vi "rethinkdb_hashlib_sha256_hmac.vi"(10 "data":string="The quick brown fox jumps over the lazy dog", 11 "key":string="key") -> (3 "sha256":u32[](array[numeric]) format="%08x")   [LabVIEW 2017]
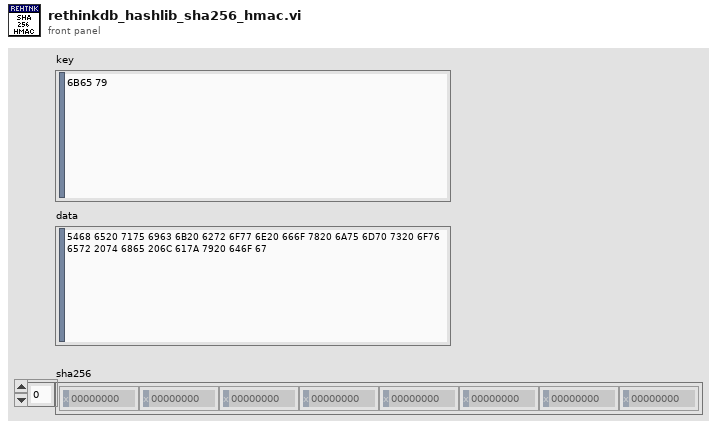
[diagram p1: front panel]
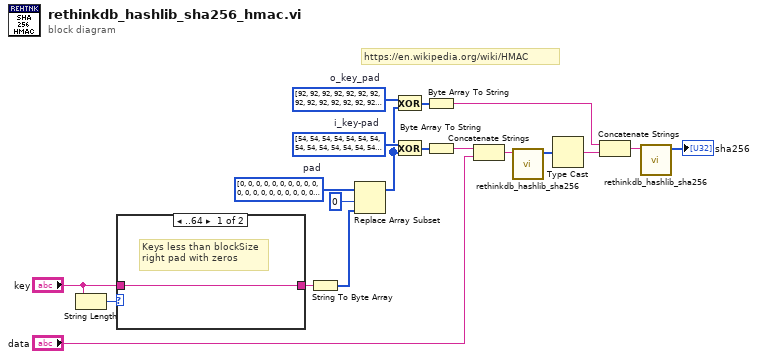
[diagram p0: block diagram]
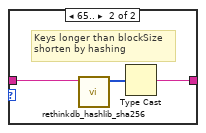
[diagram p2: hidden frame]
diagram:
  w8 = u8[] [0, 0, 0, 0, 0, 0, 0, 0, 0, 0, 0, 0, 0, 0, 0, 0, 0, 0, 0, 0, 0, 0, 0, 0, 0, 0, 0, 0, 0, 0, 0, 0, 0, 0, 0, 0, 0, 0, 0, 0, 0, 0, 0, 0, 0, 0, 0, 0, 0, 0, 0, 0, 0, 0, 0, 0, 0, 0, 0, 0, 0, 0, 0, 0]  # pad
  w10 = u8[] [92, 92, 92, 92, 92, 92, 92, 92, 92, 92, 92, 92, 92, 92, 92, 92, 92, 92, 92, 92, 92, 92, 92, 92, 92, 92, 92, 92, 92, 92, 92, 92, 92, 92, 92, 92, 92, 92, 92, 92, 92, 92, 92, 92, 92, 92, 92, 92, 92, 92, 92, 92, 92, 92, 92, 92, 92, 92, 92, 92, 92, 92, 92, 92]  # o_key_pad
  w9 = u8[] [54, 54, 54, 54, 54, 54, 54, 54, 54, 54, 54, 54, 54, 54, 54, 54, 54, 54, 54, 54, 54, 54, 54, 54, 54, 54, 54, 54, 54, 54, 54, 54, 54, 54, 54, 54, 54, 54, 54, 54, 54, 54, 54, 54, 54, 54, 54, 54, 54, 54, 54, 54, 54, 54, 54, 54, 54, 54, 54, 54, 54, 54, 54, 54]  # i_key-pad
  # "https://en.wikipedia.org/wiki/HMAC"
  n1 = String Length(string="key") -> (length=w12:i32)
  n2 = case shown="..64" w12 {
    tunnel: "key" -> [w20 w21]
    tunnel: [w20 w22] -> w7
    frame ..64 {
      # "Keys less than blockSize\nright pad with zeros"
    }
    frame 65.. {
      # "Keys longer than blockSize\nshorten by hashing"
      n3 = call "rethinkdb_hashlib_sha256.vi"("data"=w21) -> ("sha256"=w23:u32[])  [unwired: 10 in]
      n4 = Type Cast(x=w23) -> (*(type *) &x=w22:string)  [unwired: 1 in]
    }
  }
  n5 = String To Byte Array(string=w7) -> (unsigned byte array=w6:u8[])
  n6 = Replace Array Subset(array=w8, new element=w6, index=0) -> (w5:u8[])
  n7 = Exclusive Or(1:w5, 2:w10) -> (0:w15:u8[])
  n8 = Exclusive Or(1:w5, 2:w9) -> (0:w19:u8[])
  n9 = Byte Array To String(unsigned byte array=w15) -> (string=w2:string)
  n10 = Byte Array To String(unsigned byte array=w19) -> (string=w18:string)
  n11 = Concatenate Strings(w18, "data") -> (w16:string)
  n12 = call "rethinkdb_hashlib_sha256.vi"("data"=w16) -> ("sha256"=w14:u32[])  [unwired: 10 in]
  n13 = Type Cast(x=w14) -> (*(type *) &x=w3:string)  [unwired: 1 in]
  n14 = Concatenate Strings(w2, w3) -> (w1:string)
  n15 = call "rethinkdb_hashlib_sha256.vi"("data"=w1) -> ("sha256"=→"sha256":u32[])  [unwired: 10 in]
